vi "Fpga-Mix_COL-U32.vi"(11 "Numeric in":u32) -> (3 "Numeric out":u32)   [LabVIEW 2017]
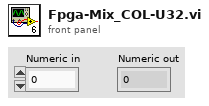
[diagram p1: front panel]
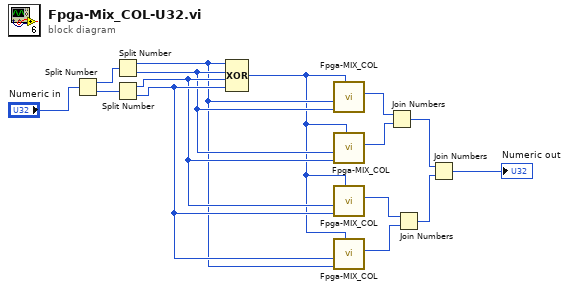
[diagram p0: block diagram]
diagram:
  n1 = Split Number(x="Numeric in") -> (hi(x)=w3:u16, lo(x)=w2:u16)
  n2 = Split Number(x=w3) -> (hi(x)=w5:u8, lo(x)=w6:u8)
  n3 = Split Number(x=w2) -> (hi(x)=w7:u8, lo(x)=w8:u8)
  n4 = Compound Arithmetic op=XOR(w5, w6, w7, w8) -> (w4:u8)
  n5 = call "Fpga-MIX_COL.vi"("Tmp"=w4, "state[i][y]"=w6, "state[i][x]"=w5) -> ("state[i][x]"=w11:u8)  [unwired: 8 in]
  n6 = call "Fpga-MIX_COL.vi"("Tmp"=w4, "state[i][y]"=w7, "state[i][x]"=w6) -> ("state[i][x]"=w12:u8)  [unwired: 8 in]
  n7 = call "Fpga-MIX_COL.vi"("Tmp"=w4, "state[i][y]"=w8, "state[i][x]"=w7) -> ("state[i][x]"=w13:u8)  [unwired: 8 in]
  n8 = call "Fpga-MIX_COL.vi"("Tmp"=w4, "state[i][y]"=w5, "state[i][x]"=w8) -> ("state[i][x]"=w14:u8)  [unwired: 8 in]
  n9 = Join Numbers(hi=w11, lo=w12) -> ((hi.lo)=w9:u16)
  n10 = Join Numbers(hi=w13, lo=w14) -> ((hi.lo)=w10:u16)
  n11 = Join Numbers(hi=w9, lo=w10) -> ((hi.lo)=→"Numeric out":u32)
